vi "copy template source to new location.vi"(8 "error in":errorcluster, 10 "destination directory (default data directory if empty)":path=path "C:/Users/nitest/Documents/LabVIEW Data", 11 "custom device name":string) -> (0 "error out":errorcluster, 3 "custom device path out":path)   [LabVIEW 2020, in "Template Tool.lvlib"]
uses:
  Template Tool.lvlib
  Template Tool Global.vi
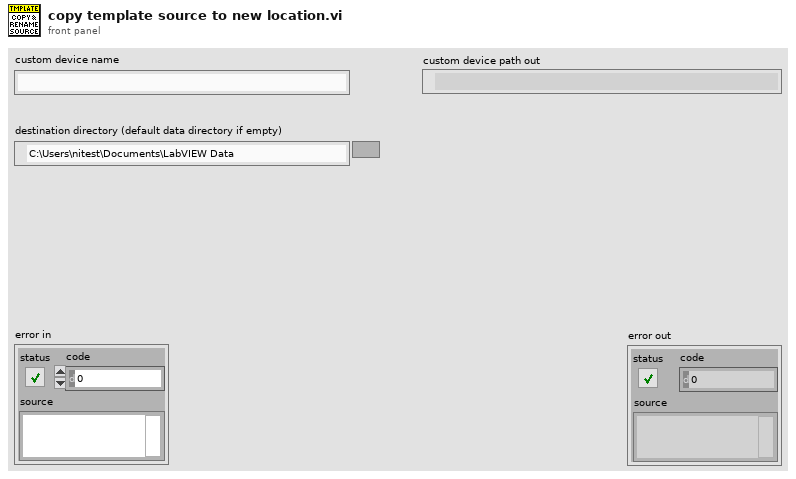
[diagram p1: front panel]
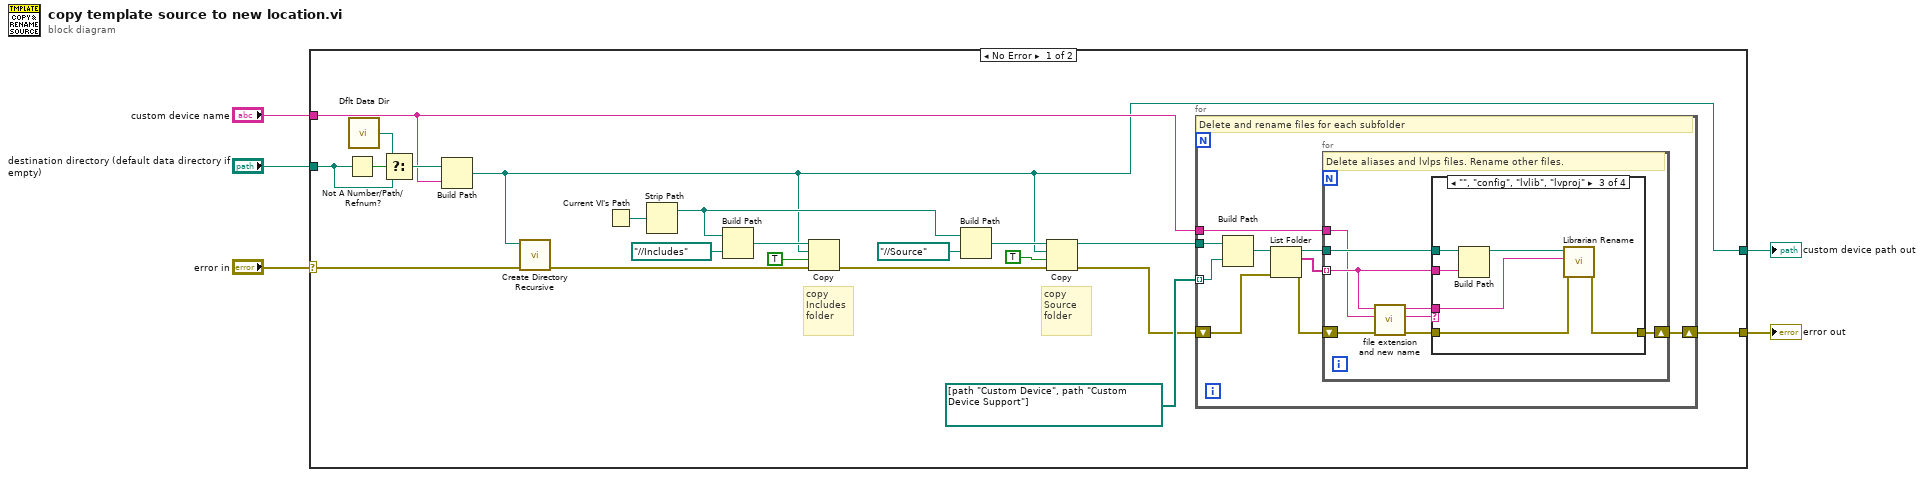
[diagram p0: block diagram]
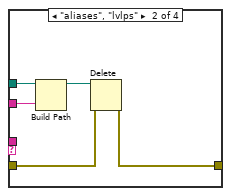
[diagram p3: hidden frame]
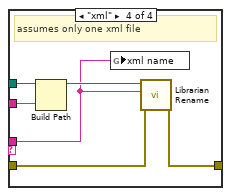
[diagram p4: hidden frame]
diagram:
  n1 = case shown="No Error" "error in" {
    selector: "error in" -> [w7 w62]
    tunnel: "destination directory (default data directory if empty)" -> [w23 _]
    tunnel: [w21 w62] -> w4
    tunnel: [w6 _] -> w3
    tunnel: "custom device name" -> [w17 _]
    frame No Error {
      # "copy Source folder"
      # "copy Includes folder"
      n2 = Not A Number/Path/Refnum?(number/path/refnum=w23) -> (NaN/Path/Refnum?=w25:bool)
      n3 = call <vilib>:"Dflt Data Dir.vi"() -> ("App:Default Data Directory"=w24:path)
      n4 = Select(t=w24, s=w25, f=w23) -> (s? t:f=w18:path)
      n5 = Build Path(base path=w18, name or relative path=w17) -> (appended path=w6:path)
      n6 = call <vilib>:"Create Directory Recursive.vi"("error in (no error)"=w7, "directory"=w6) -> ("error out"=w8:errorcluster)  [unwired: 3 in, 2 out]
      n7 = Current VI's Path() -> (path=w26:path)
      n8 = Strip Path(path=w26) -> (stripped path=w11:path)  [unwired: 1 out]
      n9 = Build Path(base path=w11, name or relative path=path "../../Includes") -> (appended path=w16:path)
      n10 = Copy(8:w8, 9:TRUE ("overwrite (F)"), 10:w6, 11:w16) -> (0:w12:errorcluster)  [unwired: 1 in, 2 out]
      n11 = Build Path(base path=w11, name or relative path=path "../../Source") -> (appended path=w15:path)
      n12 = Copy(8:w12, 9:TRUE ("overwrite (F)"), 10:w6, 11:w15) -> (0:w10:errorcluster, 3:w9:path)  [unwired: 1 in, 1 out]
      n13 = for {
        tunnel: w17 -> [w32]
        tunnel: w9 -> [w29]
        shift-right: [w31] -> w21
        shift-left: w10 -> [w35]
        tunnel: path[] [path "Custom Device", path "Custom Device Support"] -> [w27] mode=indexing
        # "Delete and rename files for each subfolder"
        n14 = Build Path(base path=w29, name or relative path=w27) -> (appended path=w30:path)
        n15 = List Folder(path=w30, error in=w35) -> (path out=w28:path, filenames=w34:string[], error out=w33:errorcluster)  [unwired: 2 in, 1 out]
        n16 = for {
          tunnel: w28 -> [w43]
          tunnel: w34 -> [w41] mode=indexing
          shift-right: [w42] -> w31
          shift-left: w33 -> [w37]
          tunnel: w32 -> [w38]
          # "Delete aliases and lvlps files. Rename other files."
          n17 = call "file extension and new name.vi"("error in"=w37, "custom device name"=w38, "filename"=w41) -> ("error out"=w36:errorcluster, "extension"=w39:string, "new filename"=w40:string)  [unwired: 6 in]
          n18 = case shown="\"\", \"config\", \"lvlib\", \"lvproj\"" w39 {
            tunnel: w43 -> [_ w48 w55 w61]
            tunnel: w41 -> [_ w47 w54 w60]
            tunnel: w36 -> [w44 w46 w53 w59]
            tunnel: [w44 w45 w52 w58] -> w42
            tunnel: w40 -> [_ _ w50 w56]
            frame Default {
            }
            frame "aliases", "lvlps" {
              n19 = Build Path(base path=w48, name or relative path=w47) -> (appended path=w49:path)
              n20 = Delete(path (use dialog)=w49, error in=w46) -> (error out=w45:errorcluster)  [unwired: 3 in, 2 out]
            }
            frame "", "config", "lvlib", "lvproj" {
              n21 = Build Path(base path=w55, name or relative path=w54) -> (appended path=w51:path)
              n22 = call <vilib>:"Librarian Rename.vi"("error in (no error)"=w53, "new name"=w50, "path"=w51) -> ("error out"=w52:errorcluster)  [unwired: 7 in, 1 out]
            }
            frame "xml" {
              # "assumes only one xml file"
              n23 = Build Path(base path=w61, name or relative path=w60) -> (appended path=w57:path)
              n24 = global write "Template Tool Global.vi" "xml name"(w56) -> ()
              n25 = call <vilib>:"Librarian Rename.vi"("error in (no error)"=w59, "new name"=w56, "path"=w57) -> ("error out"=w58:errorcluster)  [unwired: 7 in, 1 out]
            }
          }
        }
      }
    }
    frame Error {
    }
  }
  "custom device path out" <- w3
  "error out" <- w4
